vi "Main UI Variables.vi"() -> (2 "Main UI.vi":T3={"Error"={"status"=FALSE, "code"=0, "source"=""}, "Exit"=FALSE, "LocalQ"={"LocalName"="", "LocalEvent"="", "LocalData"=variant}, "Q-LowLevel"={"Q-LowLevel Name"="", "Q-LowLevel Order"="", "Q-LowLevel Data"=variant}, "Ref"={"VIRef"=refnum, "Tree"=refnum}, "Threads"={"Cfg"="", "Disp"="", "VCH"="", "Data"="", "SavePara"=""}, "InsertUI"="", "Path"={"System Config"=path "", "User Archives"=path "", "Error Log"=path "", "DynaThreads"=path "", "TreePNG"=path ""}, "User Archives"={"User Archives"=[{"User Name"="Admin", "Code"="123456", "Ability"=enum."Administrator", "Last Log Time"=timestamp(3476160307.20119 s since 1904-01-01)}, {"User Name"="Liusj", "Code"="123456", "Ability"=enum."Operator", "Last Log Time"=timestamp(3476160734.0536046 s since 1904-01-01)}], "Current User"=-1}, "FailedThreads"=[], "Buffers"={"DataBuf"=refnum}, "DevName"=""})   [LabVIEW 2016]
uses:
  Utility/Sys Paths.ctl
  Utility/User Login_Archives Data Structure.ctl
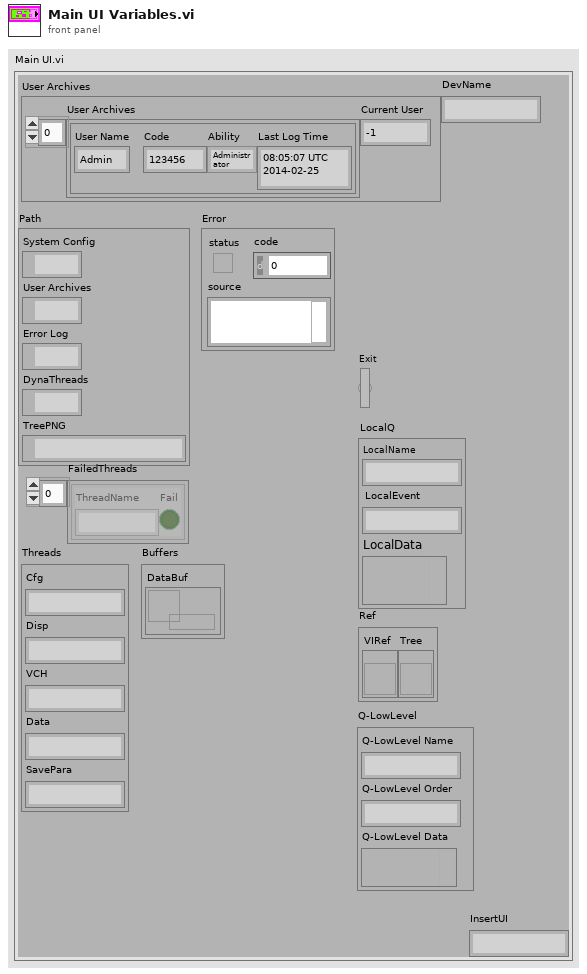
[diagram p1: front panel]
types:
  T1 = typedef "Sys Paths.ctl" = cluster{"System Config":path, "User Archives":path, "Error Log":path, "DynaThreads":path, "TreePNG":path}
  T2 = typedef "User Login_Archives Data Structure.ctl" = cluster{"User Archives":cluster{"User Name":string, "Code":string, "Ability":enum16{"Administrator", "Operator"}, "Last Log Time":timestamp}[], "Current User":i32}
  T3 = cluster{"Error":errorcluster, "Exit":bool, "LocalQ":cluster{"LocalName":string, "LocalEvent":string, "LocalData":variant}, "Q-LowLevel":cluster{"Q-LowLevel Name":string, "Q-LowLevel Order":string, "Q-LowLevel Data":variant}, "Ref":cluster{"VIRef":refnum<vi>, "Tree":refnum<vi>}, "Threads":cluster{"Cfg":string, "Disp":string, "VCH":string, "Data":string, "SavePara":string}, "InsertUI":string, "Path":T1, "User Archives":T2, "FailedThreads":cluster{"ThreadName":string, "Fail":bool}[], "Buffers":cluster{"DataBuf":refnum<queue>}, "DevName":string}
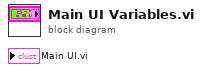
[diagram p0: block diagram]
diagram:
